vi "DAQX mod 1SDI v02.vi"(0 "resource name":refnum<k15>="PXI1Slot2", 1 "close (T)":bool=TRUE, 2 "Record Data":bool, 3 "numSamples":i32=-1, 4 "max time (s)":dbl=10.0 caption="max time", 5 "min sample rate":dbl=100000000.0, 6 "File location":path, 7 "error in":errorcluster, 8 "reference position":dbl=50.0, 9 "Additional text":string, 10 "Type of measurement":T2, 11 "Name root":string, 12 "Monitor On":bool, 13 "channel parameters":T4(array[cluster])=[{"channel name"="0", "input impedance"=0, "maximum input frequency"=30000000.0, "vertical coupling"=1, "probe attenuation"=1.0, "vertical range"=2.0, "vertical offset"=0.0, "channel enabled"=TRUE}, {"channel name"="1", "input impedance"=0, "maximum input frequency"=30000000.0, "vertical coupling"=1, "probe attenuation"=1.0, "vertical range"=2.0, "vertical offset"=0.0, "channel enabled"=TRUE}] {"input impedance" items=["1 mega ohm"=0, "50 ohms"=2]; "vertical coupling" items=["AC", "DC", "Ground"]}, 15 "reset sn":bool) -> (18 "wfm out":waveform(dbl)[](array[waveform]), 19 "file saved":path, 22 "Parameters values file":string, 24 "actualSamples 0":i32, 26 "actualSamples 1":i32, 27 "error out":errorcluster caption="error out final")   [LabVIEW 2013]
doc: "Configures and acquires data from an NI-SCOPE high-speed digitizer.\n--------------------\n\nThis Express VI is configured as follows:\n\nDevice: PXI1Slot2 (PXI-5122)\nSample Rate (S/s): 100M\nRecord length: 2k\nAcquisition Mode: N Samples\nChannel 0\n - Range (V): 2\n - Offset (V): 0\n - Probe attenuation: 1\n - Coupling: \n - Input impedence: 1 \n - Bandwidth (Hz): 0\nChannel 1\n - Range (V): 2\n - Offset (V): 0\n - Probe attenuation: 1\n - Coupling: \n - Input impedence: 1 \n - Bandwidth (Hz): 0\nImmediate"
uses:
  <instrlib>/niScope/Controls/niScope vertical coupling.ctl
  Strict Type Defs/type_meas_enum.ctl
  <instrlib>/niScope/Controls/niScope timestamp type.ctl
  <instrlib>/niScope/Acquire/Fetch/niScope Multi Fetch Binary 16.vi
  <instrlib>/niScope/Configure/Trigger/niScope Configure Trigger Immediate.vi
  Global VIs/shotnoise.vi
  <instrlib>/niScope/Acquire/Fetch/niScope Multi Fetch WDT.vi
panel:
  out "Chan 1 params":T1
  out "Chan 0 params":T1
  out "file location into parameter files":path
  out "size(s)":i32
  out "actual sample rate":dbl
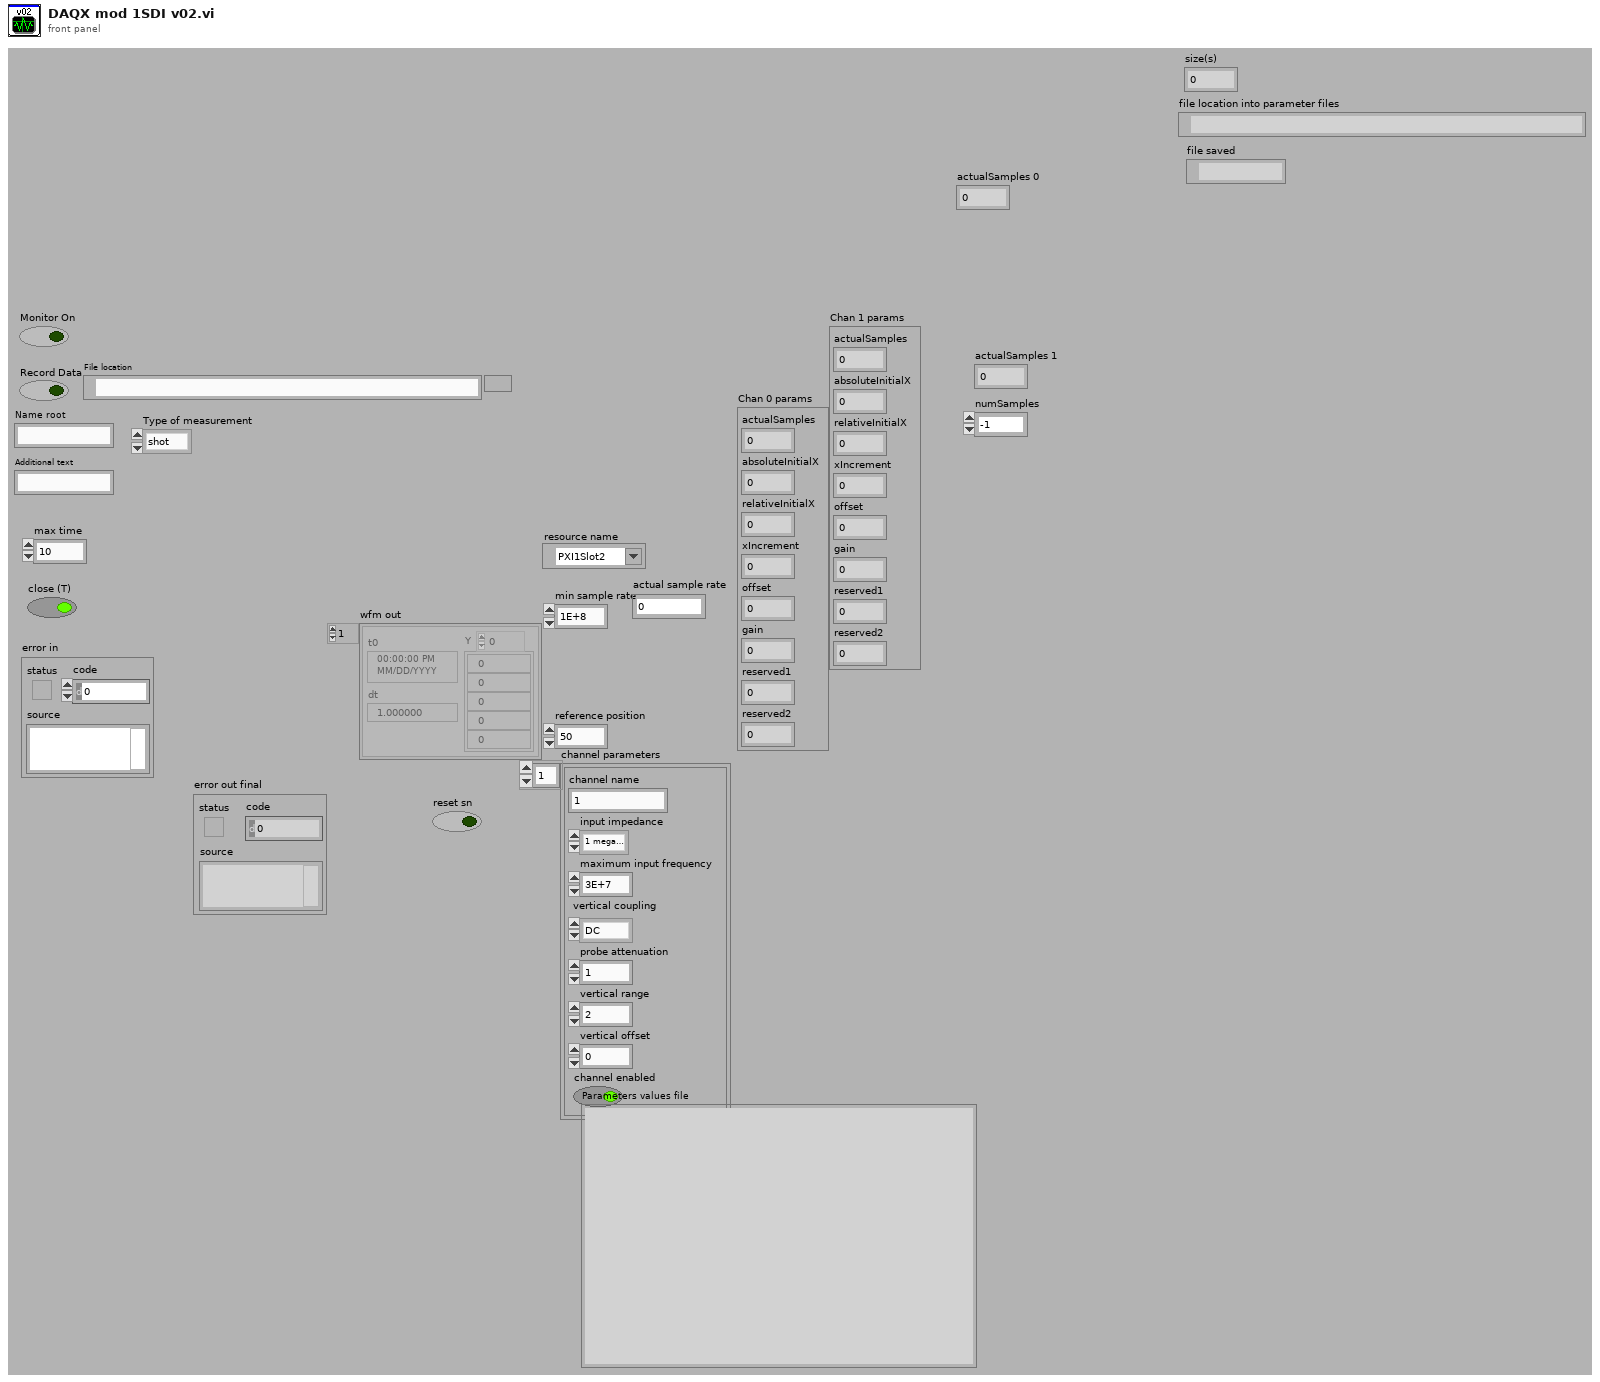
[diagram p1: front panel]
types:
  T1 = cluster{"actualSamples":i32, "absoluteInitialX":dbl, "relativeInitialX":dbl, "xIncrement":dbl, "offset":dbl, "gain":dbl, "reserved1":dbl, "reserved2":dbl}
  T2 = typedef "type_meas_enum.ctl" = enum16{"shot", "x", "p", "electronic"}
  T3 = typedef "niScope vertical coupling.ctl" = i32
  T4 = cluster{"channel name":string, "input impedance":u32, "maximum input frequency":dbl, "vertical coupling":T3, "probe attenuation":dbl, "vertical range":dbl, "vertical offset":dbl, "channel enabled":bool}[]
  T5 = typedef "niScope timestamp type.ctl" = i32
  T6 = cluster{"actualSamples":i32, "absoluteInitialX":dbl, "relativeInitialX":dbl, "xIncrement":dbl, "offset":dbl, "gain":dbl, "reserved1":dbl, "reserved2":dbl}[]
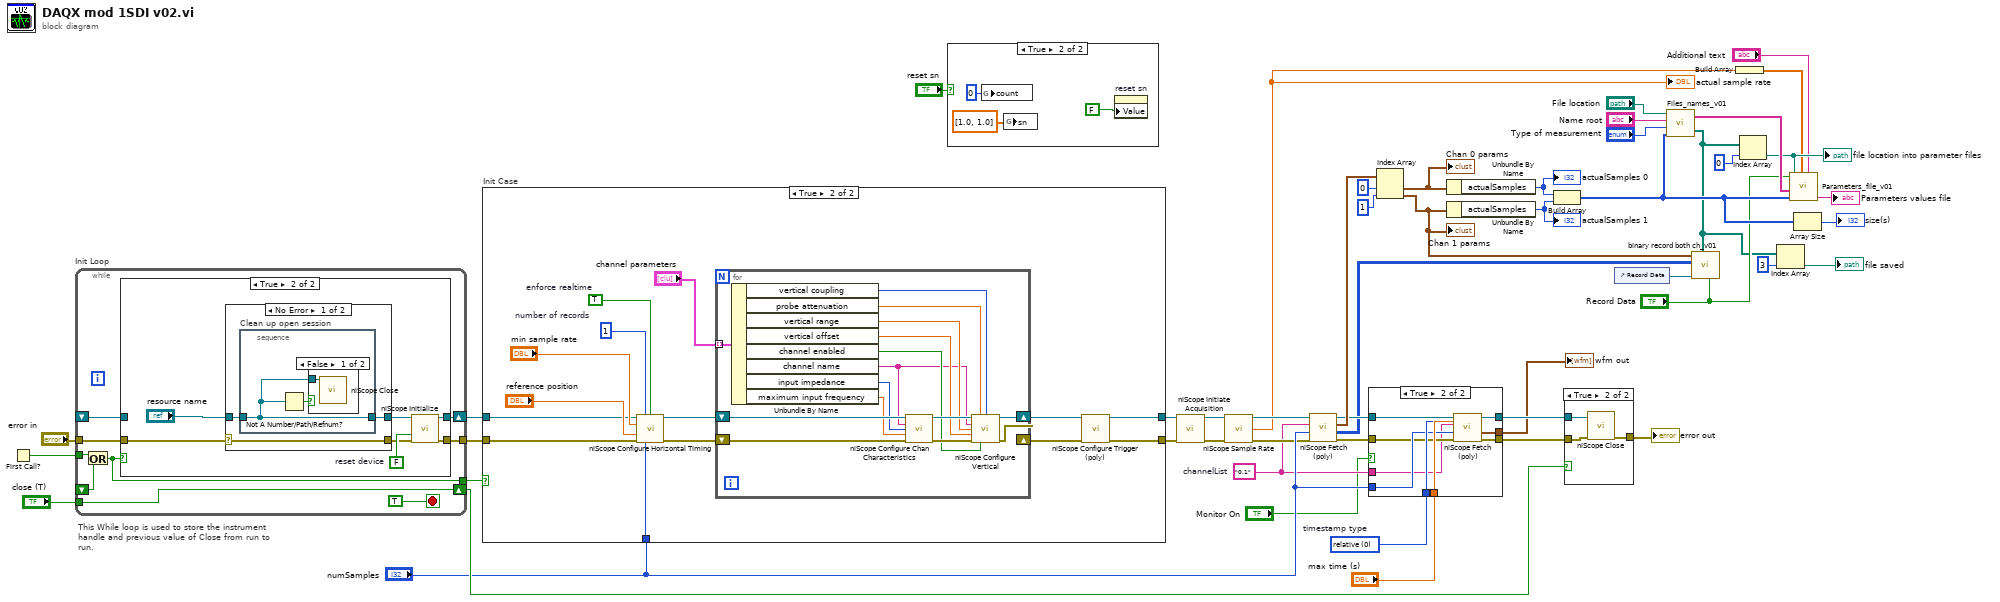
[diagram p0: block diagram]
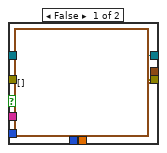
[diagram p2: hidden frame]
diagram:
  w6 = "0,1"  # channelList
  w46 = T5 0 items=["relative", "absolute"]  # timestamp type
  # "This While loop is used to store the instrument handle and previous value of Close from run to run."
  n1 = First Call?() -> (First Call?: T/F=w45:bool)
  n2 = while "Init Loop" {
    tunnel: w45 -> [w59]
    shift-right: [w58] -> w41
    shift-left: _ -> [w55]
    tunnel: "close (T)" -> [w58]
    shift-right: [w57] -> w44
    shift-left: _ -> [w56]
    tunnel: [w53] -> w43
    tunnel: "error in" -> [w52]
    tunnel: [w51] -> w42
    stop <- TRUE ("stopInit") stop-if-true
    n3 = Or(x=w59, y=w55) -> (x .or. y?=w51:bool)
    n4 = case "Select_Init" shown="True" w51 {
      tunnel: [w61 w66] -> w57
      tunnel: w56 -> [w61 _]
      tunnel: [w60 w65] -> w53
      tunnel: w52 -> [w60 w64]
      frame False {
      }
      frame True {
        w67 = FALSE  # reset device
        n5 = case shown="No Error" w64 {
          selector: w64 -> [w69 w75]
          tunnel: [w71 w76] -> w68
          tunnel: "resource name" -> [w70 w76]
          tunnel: [w69 w75] -> w63
          frame No Error {
            n6 = stacked-sequence "Clean up open session" {
              tunnel: w70 -> [w72]
              tunnel: [w72] -> w71
              frame #0 {
                n7 = Not A Number/Path/Refnum?(number/path/refnum=w72) -> (NaN/Path/Refnum?=w73:bool)
                n8 = case shown="False" w73 {
                  tunnel: w72 -> [w74 _]
                  frame False {
                    n9 = call <instrlib>:"niScope Close.vi"("instrument handle"=w74) -> ()  [unwired: 1 in, 14 out]
                  }
                  frame True {
                  }
                }
              }
            }
          }
          frame Error {
          }
        }
        n10 = call <instrlib>:"niScope Initialize.vi"("resource name"=w68, "reset device"=w67, "error in"=w63) -> ("instrument handle"=w66:refnum<k15>, "error out"=w65:errorcluster)  [unwired: 2 in, 9 out]
      }
    }
  }
  n11 = case "Init Case" shown="True" w42 {
    tunnel: w43 -> [w77 w83]
    tunnel: [w77 w85] -> w48
    tunnel: [w78 w86] -> w47
    tunnel: w44 -> [w78 w84]
    tunnel: "numSamples" -> [_ w79]
    frame False {
    }
    frame True {
      w91 = 1  # number of records
      w92 = TRUE  # enforce realtime
      n12 = call <instrlib>:"niScope Configure Horizontal Timing.vi"("instrument handle"=w84, "number of records"=w91, "enforce realtime"=w92, "min sample rate"="min sample rate", "reference position"="reference position", "error in"=w83, "min record length"=w79) -> ("instrument handle out"=w87:refnum<k15>, "error out"=w88:errorcluster)  [unwired: 7 out]
      n13 = for {
        shift-right: [w95] -> w80
        shift-left: w88 -> [w107]
        shift-right: [w94] -> w81
        shift-left: w87 -> [w106]
        tunnel: "channel parameters" -> [w103] mode=indexing
        n14 = Unbundle By Name(w103) -> ("vertical coupling"=w100:T3, "probe attenuation"=w99:dbl, "vertical range"=w98:dbl, "vertical offset"=w97:dbl, "channel enabled"=w96:bool, "channel name"=w93:string, "input impedance"=w101:u32, "maximum input frequency"=w102:dbl)
        n15 = call <instrlib>:"niScope Configure Chan Characteristics.vi"("instrument handle"=w106, "channels"=w93, "input impedance"=w101, "maximum input frequency"=w102, "error in"=w107) -> ("instrument handle out"=w105:refnum<k15>, "error out"=w104:errorcluster)  [unwired: 9 out]
        n16 = call <instrlib>:"niScope Configure Vertical.vi"("instrument handle"=w105, "probe attenuation"=w99, "vertical coupling"=w100, "channels"=w93, "vertical range"=w98, "vertical offset"=w97, "error in"=w104, "channel enabled"=w96) -> ("instrument handle out"=w94:refnum<k15>, "error out"=w95:errorcluster)  [unwired: 6 out]
      }
      n17 = call-poly <instrlib>:"niScope Configure Trigger (poly).vi"("instrument handle"=w81, "error in"=w80) -> ("instrument handle out"=w86:refnum<k15>, "error out"=w85:errorcluster)  [unwired: 12 out]
    }
  }
  n18 = case shown="True" "reset sn" {
    frame False {
    }
    frame True {
      n19 = global write "shotnoise.vi" "count"(i64 0 ("count")) -> ()
      n20 = global write "shotnoise.vi" "sn"(dbl[] [1.0, 1.0] ("sn")) -> ()
      n21 = property on="reset sn" class="Bool (strict)"("Value"=FALSE ("reset sn")) -> ()  [unwired: 2 in, 2 out]
    }
  }
  n22 = call <instrlib>:"niScope Initiate Acquisition.vi"("instrument handle"=w47, "error in"=w48) -> ("instrument handle out"=w38:refnum<k15>, "error out"=w37:errorcluster)  [unwired: 12 out]
  n23 = call <instrlib>:"niScope Sample Rate.vi"("instrument handle"=w38, "error in"=w37) -> ("instrument handle out"=w33:refnum<k15>, "actual sample rate"=w5:dbl, "error out"=w32:errorcluster)  [unwired: 11 out]
  "actual sample rate" <- w5
  n24 = call-poly <instrlib>:"niScope Fetch (poly).vi"("error in"=w32, "numSamples"="numSamples", "channels"=w6, "instrument handle"=w33) -> ("error out"=w15:errorcluster, "wfm"=w8:i16[][], "wfm info"=w31:T6, "instrument handle out"=w16:refnum<k15>)  [unwired: 1 in, 3 out]
  n25 = case shown="True" "Monitor On" {
    tunnel: "max time (s)" -> [_ w122]
    tunnel: w46 -> [_ w121]
    tunnel: [w112 w120] -> w36
    tunnel: "numSamples" -> [_ w119]
    tunnel: w16 -> [w112 w118]
    tunnel: w15 -> [w113 w117]
    tunnel: [w113 w116] -> w13
    tunnel: [waveform(dbl)[] [] ("wfm") w115] -> w12
    tunnel: w6 -> [_ w114]
    frame False {
    }
    frame True {
      n26 = call-poly <instrlib>:"niScope Fetch (poly).vi"("timestamp Type"=w121, "timeout"=w122, "error in"=w117, "numSamples"=w119, "channels"=w114, "instrument handle"=w118) -> ("error out"=w116:errorcluster, "wfm"=w115:waveform(dbl)[], "instrument handle out"=w120:refnum<k15>)  [unwired: 3 out]
    }
  }
  "wfm out" <- w12
  n27 = Index Array(array=w31, index #1=0 ("index"), index #2=1 ("index")) -> (element #1=w28:T1, element #2=w9:T1)
  "Chan 0 params" <- w28
  "Chan 1 params" <- w9
  n28 = Unbundle By Name(w28) -> ("actualSamples"=w27:i32)
  "actualSamples 0" <- w27
  n29 = Unbundle By Name(w9) -> ("actualSamples"=w11:i32)
  "actualSamples 1" <- w11
  n30 = Build Array(w27, w11) -> (w18:i32[])
  n31 = case shown="True" w41 {
    tunnel: w13 -> [w123 w126]
    tunnel: [w123 w125] -> w50
    tunnel: w36 -> [_ w124]
    frame False {
    }
    frame True {
      n32 = call <instrlib>:"niScope Close.vi"("instrument handle"=w124, "error in"=w126) -> ("error out"=w125:errorcluster)  [unwired: 13 out]
    }
  }
  "error out" <- w50
  n33 = control-ref of="Record Data"() -> (w10:refnum<vi>)
  n34 = call "Files_names_v01.vi"("actualSamples\narray"=w18, "Type of\nmeasurement"="Type of measurement", "Name root"="Name root", "File location"="File location") -> ("Files path array"=w3:path[], "Files name array"=w23:string[])
  n35 = call "binary record both ch_v01.vi"("Record"="Record Data", "Files path array"=w3, "reference"=w10, "wfm"=w8, "Chan 1 params"=w9) -> ()  [unwired: 7 in]
  n36 = Build Array(w5) -> (w19:dbl[])
  n37 = Index Array(array=w3, index=0) -> (element=w21:path)
  "file location into parameter files" <- w21
  n38 = Index Array(array=w3, index=3) -> (element=→"file saved":path)
  n39 = call "Parameters_file_v01.vi"("Additional text"="Additional text", "actual sample rate array"=w19, "actualSamples array"=w18, "Files name array"=w23, "File location"=w21, "Record"="Record Data") -> ("Full text"=→"Parameters values file":string)  [unwired: 3 in]
  n40 = Array Size(array=w18) -> (size(s)=→"size(s)":i32)
